vi "GPIO Bank Override.vi"(0 "gpio bank output config":T2, 11 "override gpio bank output config":T2) -> (4 "gpio bank":T1, 15 "gpio bank output enable":T1)   [LabVIEW 2020, in "GettingStarted_Common_148X_FPGA.lvlib"]
uses:
  GettingStarted_Common_148X_FPGA.lvlib
  Types/GPIO Bank Output Configuration.ctl
  <instrlib>/FlexRIO/CSI-2/v2/FPGA/Types/GPIO Bank.ctl
  <instrlib>/FlexRIO/CSI-2/v2/FPGA/NI CSI-2 API FPGA v2.lvlib
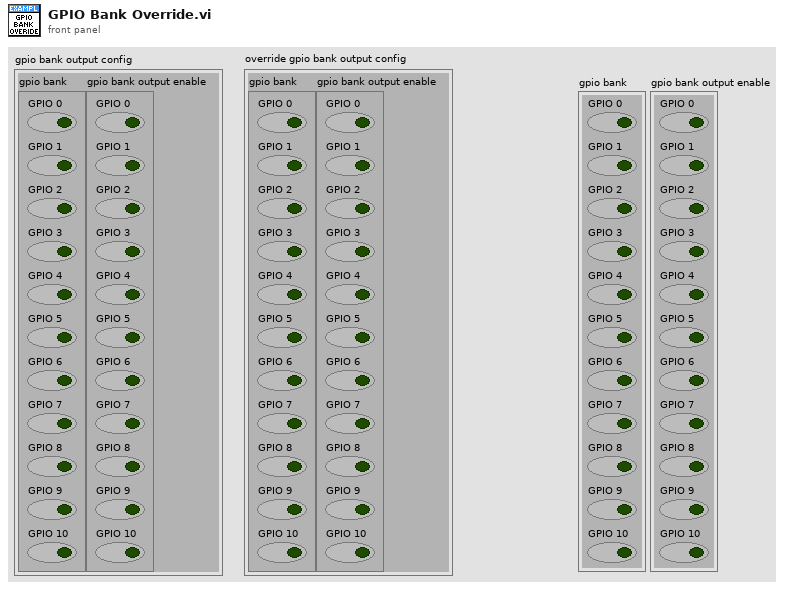
[diagram p1: front panel]
types:
  T1 = typedef "NI CSI-2 API FPGA v2.lvlib/GPIO Bank.ctl" = cluster{"GPIO 0":bool, "GPIO 1":bool, "GPIO 2":bool, "GPIO 3":bool, "GPIO 4":bool, "GPIO 5":bool, "GPIO 6":bool, "GPIO 7":bool, "GPIO 8":bool, "GPIO 9":bool, "GPIO 10":bool}
  T2 = typedef "GettingStarted_Common_148X_FPGA.lvlib/GPIO Bank Output Configuration.ctl" = cluster{"gpio bank":T1, "gpio bank output enable":T1}
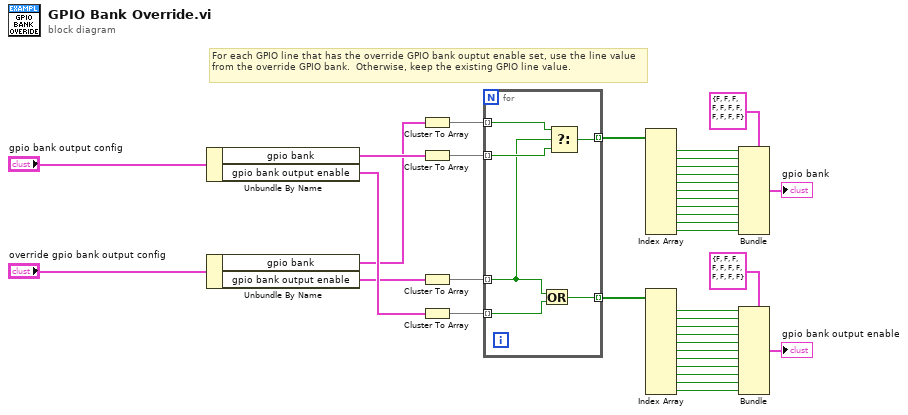
[diagram p0: block diagram]
diagram:
  # "For each GPIO line that has the override GPIO bank ouptut enable set, use the line value from the override GPIO bank.  Otherwise, keep the existing GPIO line value."
  n1 = Unbundle By Name("gpio bank output config") -> ("gpio bank"=w4:T1, "gpio bank output enable"=w6:T1)
  n2 = Unbundle By Name("override gpio bank output config") -> ("gpio bank"=w3:T1, "gpio bank output enable"=w5:T1)
  n3 = Cluster To Array(cluster=w3) -> (array=w38:bool[])
  n4 = Cluster To Array(cluster=w4) -> (array=w36:bool[])
  n5 = Cluster To Array(cluster=w5) -> (array=w37:bool[])
  n6 = Cluster To Array(cluster=w6) -> (array=w35:bool[])
  n7 = for {
    tunnel: w38 -> [w44] mode=indexing
    tunnel: w37 -> [w41] mode=indexing
    tunnel: w36 -> [w43] mode=indexing
    tunnel: w35 -> [w40] mode=indexing
    tunnel: [w42] -> w22 mode=indexing
    tunnel: [w39] -> w9 mode=indexing
    n8 = Or(x=w41, y=w40) -> (x .or. y?=w39:bool)
    n9 = Select(t=w44, s=w41, f=w43) -> (s? t:f=w42:bool)
  }
  n10 = Index Array(array=w22) -> (element #1=w24:bool, element #2=w25:bool, element #3=w26:bool, element #4=w27:bool, element #5=w28:bool, element #6=w29:bool, element #7=w30:bool, element #8=w31:bool, element #9=w32:bool, element #10=w33:bool, element #11=w34:bool)  [unwired: 11 in]
  n11 = Index Array(array=w9) -> (element #1=w11:bool, element #2=w12:bool, element #3=w13:bool, element #4=w14:bool, element #5=w15:bool, element #6=w16:bool, element #7=w17:bool, element #8=w18:bool, element #9=w19:bool, element #10=w20:bool, element #11=w21:bool)  [unwired: 11 in]
  n12 = Bundle(cluster=T1 {"GPIO 0"=FALSE, "GPIO 1"=FALSE, "GPIO 2"=FALSE, "GPIO 3"=FALSE, "GPIO 4"=FALSE, "GPIO 5"=FALSE, "GPIO 6"=FALSE, "GPIO 7"=FALSE, "GPIO 8"=FALSE, "GPIO 9"=FALSE, "GPIO 10"=FALSE} ("gpio bank output"), "GPIO 0"=w24, "GPIO 1"=w25, "GPIO 2"=w26, "GPIO 3"=w27, "GPIO 4"=w28, "GPIO 5"=w29, "GPIO 6"=w30, "GPIO 7"=w31, "GPIO 8"=w32, "GPIO 9"=w33, "GPIO 10"=w34) -> (→"gpio bank":T1)
  n13 = Bundle(cluster=T1 {"GPIO 0"=FALSE, "GPIO 1"=FALSE, "GPIO 2"=FALSE, "GPIO 3"=FALSE, "GPIO 4"=FALSE, "GPIO 5"=FALSE, "GPIO 6"=FALSE, "GPIO 7"=FALSE, "GPIO 8"=FALSE, "GPIO 9"=FALSE, "GPIO 10"=FALSE} ("gpio bank output"), "GPIO 0"=w11, "GPIO 1"=w12, "GPIO 2"=w13, "GPIO 3"=w14, "GPIO 4"=w15, "GPIO 5"=w16, "GPIO 6"=w17, "GPIO 7"=w18, "GPIO 8"=w19, "GPIO 9"=w20, "GPIO 10"=w21) -> (→"gpio bank output enable":T1)
